vi "Unregister Feed.vi"(8 "error in":errorcluster, 10 "feed name":string) -> (0 "error out":errorcluster, 2 "feed name out":string)   [LabVIEW 2014, in "NIPM_API.lvlib"]
doc: "Unregisters a feed from NI Package Manager on this computer\n\nINPUT(s)\n<b>Feed name:</b> Specifies the name of the feed to unregister.\n\nOUTPUT(s)\n<b>Feed name out:</b> Outputs the specified feed name."
uses:
  NIPM_API.lvlib
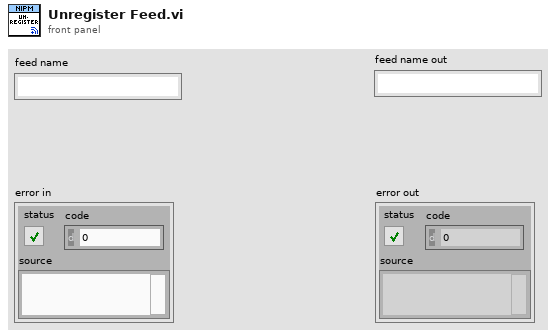
[diagram p1: front panel]
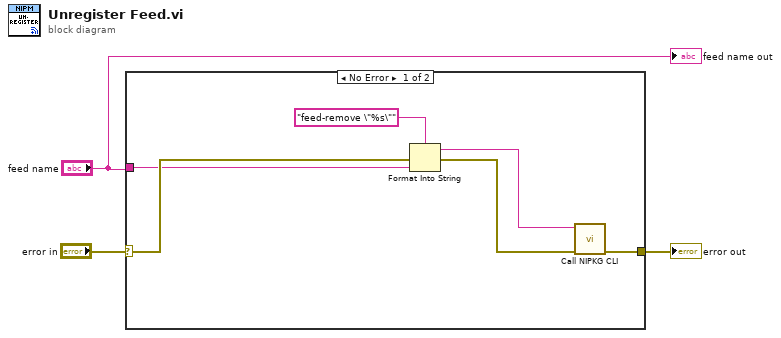
[diagram p0: block diagram]
diagram:
  n1 = case shown="No Error" "error in" {
    selector: "error in" -> [w8 w10]
    tunnel: [w5 w10] -> w2
    tunnel: "feed name" -> [w4 _]
    frame No Error {
      n2 = Format Into String(format string="feed-remove \"%s\"", error in=w8, w4) -> (resulting string=w7:string, error out=w6:errorcluster)  [unwired: 1 in]
      n3 = call "Call NIPKG CLI.vi"("error in (no error)"=w6, "command"=w7) -> ("error out"=w5:errorcluster)  [unwired: 8 in, 1 out]
    }
    frame Error {
    }
  }
  "error out" <- w2
  "feed name out" <- "feed name"
